vi "test Work Directory.vi"(8 "error in":errorcluster) -> (0 "error out":errorcluster)   [LabVIEW 2020, in "ase.test.lvlib"]
uses:
  ase.test.lvlib
  <vilib>/addons/_JKI Toolkits/Caraya/classes/Test/Test.lvclass
  ase/ase/ase.lvclass
  <vilib>/addons/_JKI Toolkits/Caraya/classes/Assert/Assert.lvclass
  <vilib>/addons/_JKI Toolkits/Caraya/classes/Assert/Assert Equal Value_Variant.vi
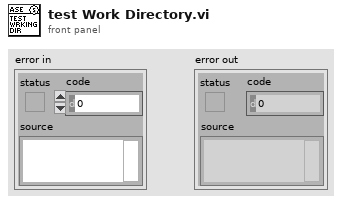
[diagram p1: front panel]
types:
  T1 = typedef "ase.lvlib/ase.lvclass/Event References.ctl" = cluster{"Standard Output":refnum<user-event>, "Standard Error":refnum<user-event>, "Did Exit":refnum<user-event>}
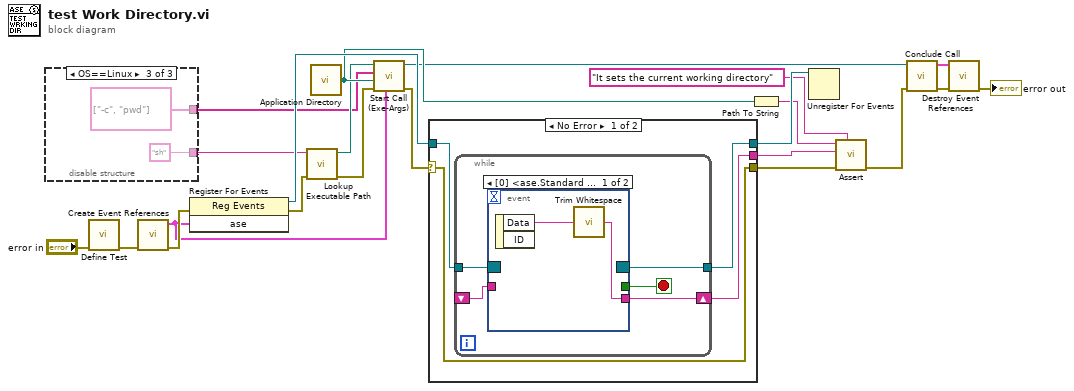
[diagram p0: block diagram]
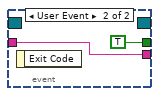
[diagram p2: hidden frame]
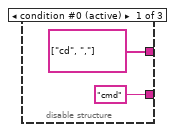
[diagram p4: hidden frame]
diagram:
  n1 = disable-structure "Conditional Disable Structure" shown="OS==Linux" {
    disable-tunnel: ["cmd" _ "sh"] -> w13
    disable-tunnel: [string[] ["cd", ","] ("Arguments (Default: Empty)") _ string[] ["-c", "pwd"] ("Arguments (Default: Empty)")] -> w1
    frame condition #0 (active) {
    }
    frame condition #1 {
    }
    frame condition #2 {
    }
  }
  n2 = call <vilib>:"Define Test.vi"("error in (no error)"="error in") -> ("error out"=w20:errorcluster)  [unwired: 9 in, 1 out]
  n3 = call "Create Event References.vi"("error in"=w20) -> ("error out"=w21:errorcluster, "ase"=w10:T1)  [unwired: 9 in]
  n4 = register-events(error in=w21, w10) -> (reference out=w18:refnum<event-registration>, error out=w3:errorcluster)  [unwired: 1 in]
  n5 = call "Lookup Executable Path.vi"("error in"=w3, "Executable Name"=w13) -> ("error out"=w2:errorcluster, "Path"=w4:path)  [unwired: 7 in, 1 out]
  n6 = call <vilib>:"Application Directory.vi"() -> ("Application Directory"=w12:path)
  n7 = call "Start Call (Exe-Args).vi"("Event References"=w10, "error in"=w2, "Working Directory (default <Not A Path> - System Default)"=w12, "Arguments (Default: Empty)"=w1, "Executable Path"=w4) -> ("error out"=w19:errorcluster, "New ASE Handle"=w9:refnum<class "ase.lvclass">)  [unwired: 5 in]
  n8 = case shown="No Error" w19 {
    selector: w19 -> [w30 w41]
    tunnel: w18 -> [w29 w40]
    tunnel: [w28 _] -> w15
    tunnel: [w27 w40] -> w17
    tunnel: [w30 w41] -> w11
    frame No Error {
      n9 = while {
        tunnel: w29 -> [w35]
        tunnel: [w33] -> w27
        shift-right: [w32] -> w28
        shift-left: _ -> [w31]
        stop <- w34 stop-if-true
        n10 = event shown="[0] <ase.Standard Output>: User Event" {
          selector: w35 -> [_ _]
          dyn-events: [_ _] -> w33
          timeout: _ -> [_ _]
          tunnel: [_ TRUE] -> w34
          tunnel: [w36 w38] -> w32
          tunnel: w31 -> [_ w38]
          event User Event {
            n11 = event-data() -> ("Data"=w37:string)  [unwired: 1 in, 1 out]
            n12 = call <vilib>:"Trim Whitespace.vi"("string"=w37) -> ("trimmed string"=w36:string)  [unwired: 1 in]
          }
          event User Event {
            n13 = event-data() -> ()  [unwired: 1 in, 1 out]
          }
        }
      }
    }
    frame Error {
    }
  }
  n14 = Path To String(path=w12) -> (string=w16:string)
  n15 = Unregister For Events(event registration refnum=w17) -> ()  [unwired: 1 in, 1 out]
  n16 = call-poly <vilib>:"Assert.vi"("Label"="It sets the current working directory", "error in (no error)"=w11, "Y"=w15, "X"=w16) -> ("error out"=w8:errorcluster)  [unwired: 6 in, 1 out]
  n17 = call "Conclude Call.vi"("error in"=w8, "ASE Handle"=w9) -> ("error out"=w7:errorcluster, "Event References"=w5:T1)  [unwired: 7 in, 1 out]
  n18 = call "Destroy Event References.vi"("error in"=w7, "Event References"=w5) -> ("error out"=→"error out":errorcluster)  [unwired: 9 in]
